vi "Cut Ratio.vi"(0 "dB On (T)":bool) -> (1 "UpperCutRatio":dbl format="%.2e", 2 "LowerCutRatio":dbl format="%.2e")   [LabVIEW 2017, in "SoundVib_Gabor.lvlib"]
uses:
  <vilib>/addons/Sound and Vibration/Order Analysis/Gabor Order Tracking/SoundVib_Gabor.lvlib
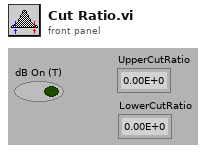
[diagram p1: front panel]
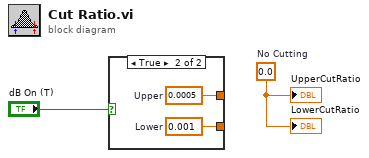
[diagram p0: block diagram]
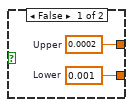
[diagram p2: hidden frame]
diagram:
  w1 = 0.0  # No Cutting
  n1 = case shown="True" "dB On (T)" {
    tunnel: [w4 w6] -> _
    tunnel: [w3 w5] -> _
    frame False {
      w3 = 0.001  # Lower
      w4 = 0.0002  # Upper
    }
    frame True {
      w5 = 0.001  # Lower
      w6 = 0.0005  # Upper
    }
  }
  "LowerCutRatio" <- w1
  "UpperCutRatio" <- w1
